vi "New ROI and Overlay Selection.vi"(8 "error in (no error)":errorcluster, 10 "ItemTag":string, 11 "IMAQ Display in":refnum<class "HIJ Vision Display.lvclass">) -> (0 "error out":errorcluster, 3 "IMAQ Display out":refnum<class "HIJ Vision Display.lvclass">)   [LabVIEW 2014, in "HIJ Vision Display.lvlib" / "HIJ Vision Display.lvclass"]
uses:
  HIJ Vision Display.lvclass
  HIJ Vision Display.lvclass/HIJ Vision Display.ctl
  Results and Overlays/Results Base/Analyze Results Base.lvclass
  Results and Overlays/Results Base/Analyze Results Base.lvclass/Analyze Results Base.ctl
  Results and Overlays/Results Base/Read Overlay_.vi
  Results and Overlays/Results Base/Write Overlay_.vi
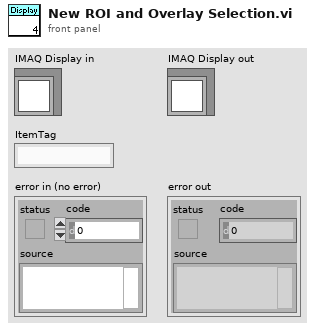
[diagram p1: front panel]
types:
  T1 = typedef "HIJ Vision Display.lvlib/HIJ Vision Display.lvclass/Named ROI.ctl" = cluster{"ROI":cluster{"Global Rectangle":i32[], "Contours":cluster{"Contour Type":u32, "ROI Type":u32, "Points":i32[]}[]}, "Name":string}
  T2 = cluster{"Global Rectangle":i32[], "Contours":cluster{"Contour Type":u32, "ROI Type":u32, "Points":i32[]}[]}
  T3 = typedef "IMAQ Image.ctl" = refnum<image>
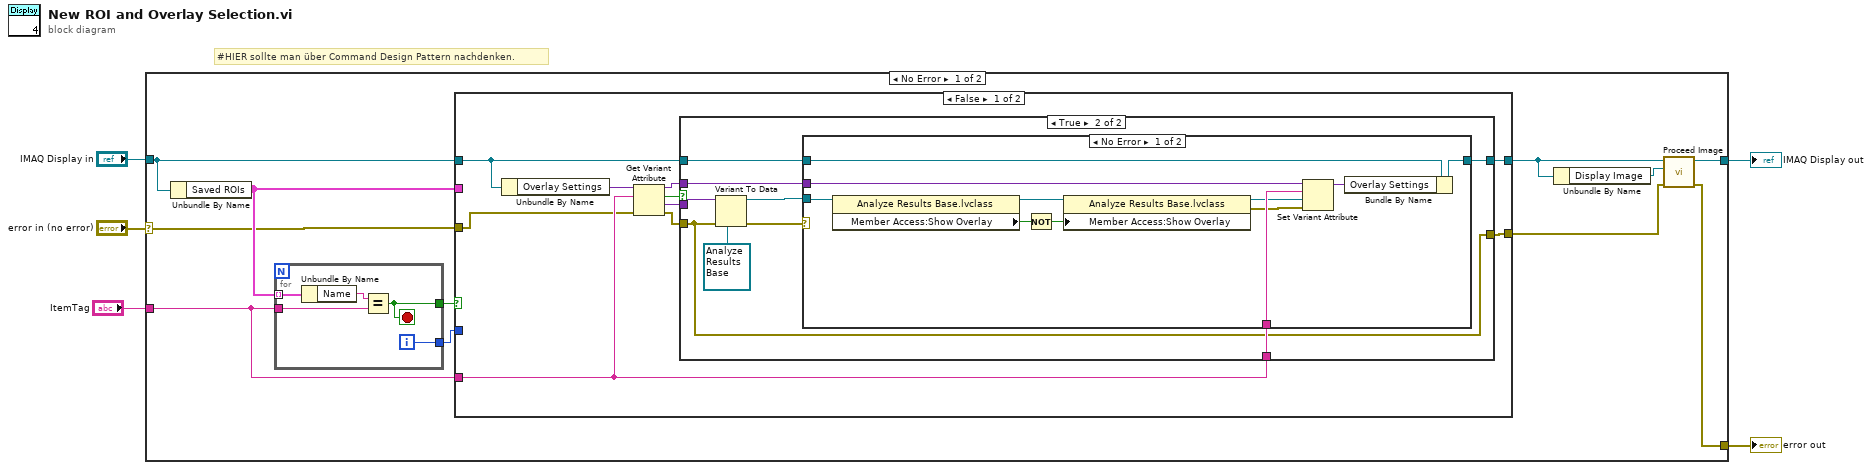
[diagram p0: block diagram]
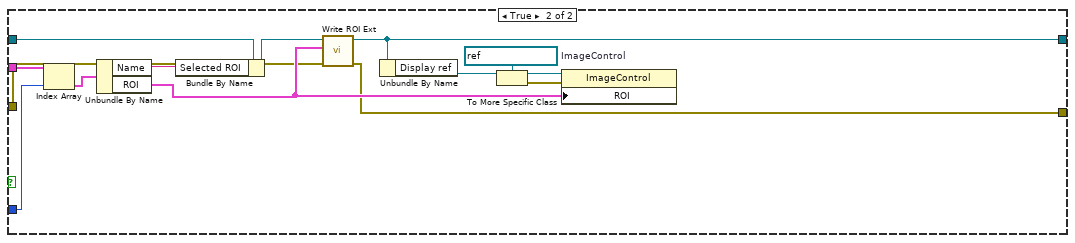
[diagram p4: hidden frame]
diagram:
  # "#HIER sollte man über Command Design Pattern nachdenken."
  n1 = case shown="No Error" "error in (no error)" {
    selector: "error in (no error)" -> [w7 w70]
    tunnel: [w8 w70] -> w4
    tunnel: [w11 w69] -> w1
    tunnel: "IMAQ Display in" -> [w12 w69]
    tunnel: "ItemTag" -> [w13 _]
    frame No Error {
      n2 = Unbundle By Name(w12) -> ("Saved ROIs"=w16:T1[])
      n3 = for {
        tunnel: w16 -> [w68] mode=indexing
        tunnel: w13 -> [w66]
        tunnel: [w65] -> w14
        tunnel: [w64] -> w15
        i -> [w64]
        stop <- w65 stop-if-true
        n4 = Unbundle By Name(w68) -> ("Name"=w67:string)
        n5 = Equal?(x=w67, y=w66) -> (x = y?=w65:bool)
      }
      n6 = case shown="False" w14 {
        tunnel: w16 -> [_ w62]
        tunnel: w15 -> [_ w63]
        tunnel: w12 -> [w21 w60]
        tunnel: w13 -> [w20 _]
        tunnel: [w19 w53] -> w10
        tunnel: w7 -> [w18 w51]
        tunnel: [w17 w50] -> w6
        frame False {
          n7 = Unbundle By Name(w21) -> ("Overlay Settings"=w26:variant)
          n8 = Get Variant Attribute(Variant=w26, name=w20, error in=w18) -> (duplicate Variant=w22:variant, found=w23:bool, value=w25:variant, error out=w24:errorcluster)  [unwired: 1 in]
          n9 = case shown="True" w23 {
            tunnel: w25 -> [_ w36]
            tunnel: w24 -> [w27 w29]
            tunnel: w22 -> [_ w33]
            tunnel: w21 -> [w28 w32]
            tunnel: w20 -> [_ w31]
            tunnel: [w28 w30] -> w19
            tunnel: [w27 w29] -> w17
            frame False {
            }
            frame True {
              n10 = Variant To Data(error in=w29, type=refnum<class "Analyze Results Base.lvclass"> refnum ("Analyze Results Base.lvclass"), Variant=w36) -> (data=w34:refnum<class "Analyze Results Base.lvclass">, error out=w35:errorcluster)
              n11 = case shown="No Error" w35 {
                tunnel: w34 -> [w47 _]
                tunnel: w33 -> [w41 _]
                tunnel: w32 -> [w43 w49]
                tunnel: w31 -> [w48 _]
                tunnel: [w38 w49] -> w30
                frame No Error {
                  n12 = property class="Analyze Results Base.lvclass"(reference=w47) -> (reference out=w46:refnum<class "Analyze Results Base.lvclass">, "Member Access:Show Overlay"=w45:bool)  [unwired: 1 in, 1 out]
                  n13 = Not(x=w45) -> (.not. x?=w44:bool)
                  n14 = property class="Analyze Results Base.lvclass"(reference=w46, "Member Access:Show Overlay"=w44) -> (reference out=w40:refnum<class "Analyze Results Base.lvclass">, error out=w42:errorcluster)  [unwired: 1 in]
                  n15 = Set Variant Attribute(Variant=w41, name=w48, value=w40, error in=w42) -> (Variant out=w39:variant)  [unwired: 2 out]
                  n16 = Bundle By Name(cluster=w43, "Overlay Settings"=w39) -> (w38:refnum<class "HIJ Vision Display.lvclass">)
                }
                frame Error {
                }
              }
            }
          }
        }
        frame True {
          w55 = refnum<vi> refnum  # ImageControl
          n17 = Index Array(array=w62, index=w63) -> (element=w61:T1)
          n18 = Unbundle By Name(w61) -> ("Name"=w59:string, "ROI"=w52:T2)
          n19 = Bundle By Name(cluster=w60, "Selected ROI"=w59) -> (w58:refnum<class "HIJ Vision Display.lvclass">)
          n20 = call "Write ROI Ext.vi"("error in (no error)"=w51, "ROI Descriptor"=w52, "IMAQ Display in"=w58) -> ("error out"=w50:errorcluster, "IMAQ Display out"=w53:refnum<class "HIJ Vision Display.lvclass">)  [unwired: 7 in]
          n21 = Unbundle By Name(w53) -> ("Display ref"=w57:refnum<vi>)
          n22 = To More Specific Class(target class=w55, reference=w57) -> (specific class reference=w56:refnum<vi>, error out=w54:errorcluster)  [unwired: 1 in]
          n23 = property class="ImageControl"(reference=w56, error in=w54, "ROI"=w52) -> ()  [unwired: 2 out]
        }
      }
      n24 = Unbundle By Name(w10) -> ("Display Image"=w9:T3)
      n25 = call "Proceed Image.vi"("error in (no error)"=w6, "Image"=w9, "IMAQ Display in"=w10) -> ("error out"=w8:errorcluster, "HIJ Vision Display out"=w11:refnum<class "HIJ Vision Display.lvclass">)  [unwired: 7 in]
    }
    frame Error {
    }
  }
  "error out" <- w4
  "IMAQ Display out" <- w1
